vi "delete mappings by seq channel.vi"(8 "error in":errorcluster, 10 "seq channel name":string, 11 "engine configuration in":refnum<class "base TBM sequencer configuration.lvclass">) -> (0 "error out":errorcluster, 3 "engine configuration out":refnum<class "base TBM sequencer configuration.lvclass">)   [LabVIEW 2014, in "base TBM sequencer configuration.lvclass"]
uses:
  base TBM sequencer configuration.lvclass
  base TBM sequencer configuration.lvclass/base TBM sequencer configuration.ctl
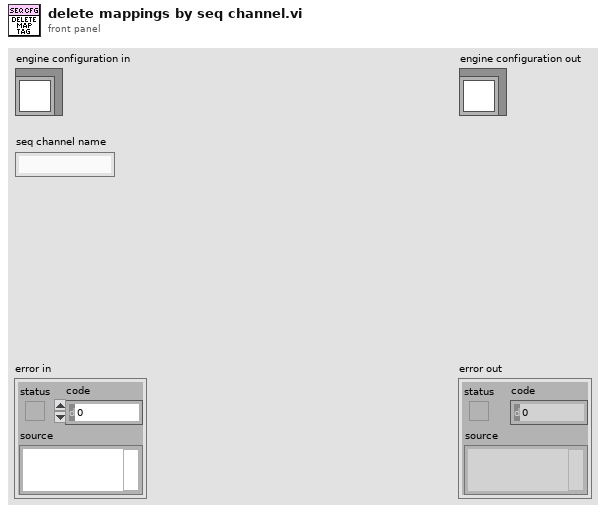
[diagram p1: front panel]
types:
  T1 = typedef "base TBM sequencer configuration.lvclass/Module Mappings.ctl" = cluster{"Owning ID":string, "Input Mappings":T2[], "Process Parameter Mappings":T2[], "Process Results Mappings":T2[], "Output Mappings":T2[]}
  T2 = typedef "tag bus.lvlib/data table.lvlib/mapping specification.ctl" = cluster{"data type":T3, "mappings":T4[]}
  T3 = typedef "tag bus.lvlib/tag descriptor.lvclass/Data Type.ctl" = enum16{"Double", "Single", "I64", "I32", "I16", "I8", "U64", "U32", "U16", "U8", "Boolean", "String", "Array of Double", "Array of Single", "Array of I64", "Array of I32", "Array of I16", "Array of I8", "Array of U64", "Array of U32", "Array of U16", "Array of U8", "Array of Boolean", "Array of String"}
  T4 = typedef "tag bus.lvlib/data table.lvlib/mapping.ctl" = cluster{"sink name":string, "source name":string}
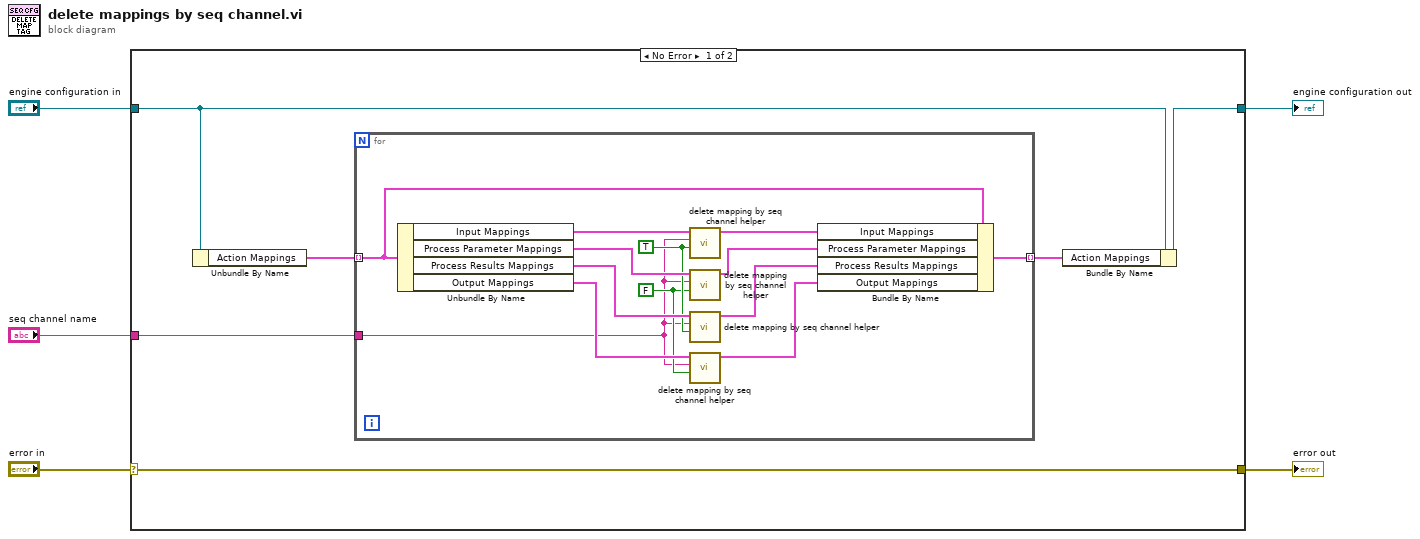
[diagram p0: block diagram]
diagram:
  n1 = case shown="No Error" "error in" {
    selector: "error in" -> [w11 w26]
    tunnel: [w11 w26] -> w4
    tunnel: [w6 w25] -> w2
    tunnel: "engine configuration in" -> [w8 w25]
    tunnel: "seq channel name" -> [w10 _]
    frame No Error {
      n2 = Unbundle By Name(w8) -> ("Action Mappings"=w9:T1[])
      n3 = for {
        tunnel: w10 -> [w18]
        tunnel: w9 -> [w17] mode=indexing
        tunnel: [w12] -> w7 mode=indexing
        w19 = FALSE
        w20 = TRUE
        n4 = Unbundle By Name(w17) -> ("Input Mappings"=w24:T2[], "Process Parameter Mappings"=w23:T2[], "Process Results Mappings"=w22:T2[], "Output Mappings"=w21:T2[])
        n5 = call "delete mapping by seq channel helper.vi"("input channel?"=w20, "channel name"=w18, "Mappings"=w24) -> ("Mappings out"=w16:T2[])  [unwired: 8 in]
        n6 = call "delete mapping by seq channel helper.vi"("input channel?"=w19, "channel name"=w18, "Mappings"=w23) -> ("Mappings out"=w15:T2[])  [unwired: 8 in]
        n7 = call "delete mapping by seq channel helper.vi"("input channel?"=w20, "channel name"=w18, "Mappings"=w22) -> ("Mappings out"=w14:T2[])  [unwired: 8 in]
        n8 = call "delete mapping by seq channel helper.vi"("input channel?"=w19, "channel name"=w18, "Mappings"=w21) -> ("Mappings out"=w13:T2[])  [unwired: 8 in]
        n9 = Bundle By Name(cluster=w17, "Input Mappings"=w16, "Process Parameter Mappings"=w15, "Process Results Mappings"=w14, "Output Mappings"=w13) -> (w12:T1)
      }
      n10 = Bundle By Name(cluster=w8, "Action Mappings"=w7) -> (w6:refnum<class "base TBM sequencer configuration.lvclass">)
    }
    frame Error {
    }
  }
  "error out" <- w4
  "engine configuration out" <- w2
